vi "Swerve Calculate Angle and Velocity.vi"(4 "Max Translation Output(0-1)":dbl=1.0, 6 "Rotation Reduction":dbl=1.0, 7 "Frame":T1={"Length"=5.0, "Width"=1020.0}, 8 "Rotation Center From Robot Center":T2, 11 "Comand Data":T7 {"Rotate(Yaw) CCW 1 CW -1" scale=1.0..-1.0; "Traverse"."Angle" scale format="%.3f"; "Traverse"."Velocity" scale=-1.0..1.0 scale format="%.1f"}) -> (3 "Swerve Request Out":T3 {"Back Right"."Angle" scale format="%.3f"; "Back Right"."Velocity" scale=-1.0..1.0 scale format="%.1f"; "Back Left"."Angle" scale format="%.3f"; "Back Left"."Velocity" scale=-1.0..1.0 scale format="%.1f"; "Front Left"."Angle" scale format="%.3f"; "Front Left"."Velocity" scale=-1.0..1.0 scale format="%.1f"; "Front Right"."Angle" scale format="%.3f"; "Front Right"."Velocity" scale=-1.0..1.0 scale format="%.1f"})   [LabVIEW 2020, in "SwerveDrive_ACT.lvlib"]
doc: "Performs the kinematics for a rectangular four wheel swerve robot with a selectable center of rotation. Swerve module #0 is located in the front right corner and the modules increment in the counter-clockwise direction."
uses:
  SwerveDrive_ACT.lvlib
  Shared Code/TypeDefs/Cluster_CMD_Direction Data.ctl
  Shared Code/TypeDefs/Cluster_Module Velocity-Direction-Rotations.ctl
  Shared Code/TypeDefs/Level_Velocity plus-minus 1.ctl
  Shared Code/TypeDefs/Dial_Compase heading unit circle CCW positive.ctl
  Type Defs/NUM_Rotate Input.ctl
  Shared Code/TypeDefs/Cluster_Swerve 4 Steer and Velocity.ctl
  Shared Code/TypeDefs/Cluster_X-Y.ctl
  Type Defs/Cluster_Length and Width.ctl
panel:
  # "\"Front\" of Robot"
  # "Right Hand Rule"
  # "X"
  # "+CCW"
  # "Y"
  # "(0,0)"
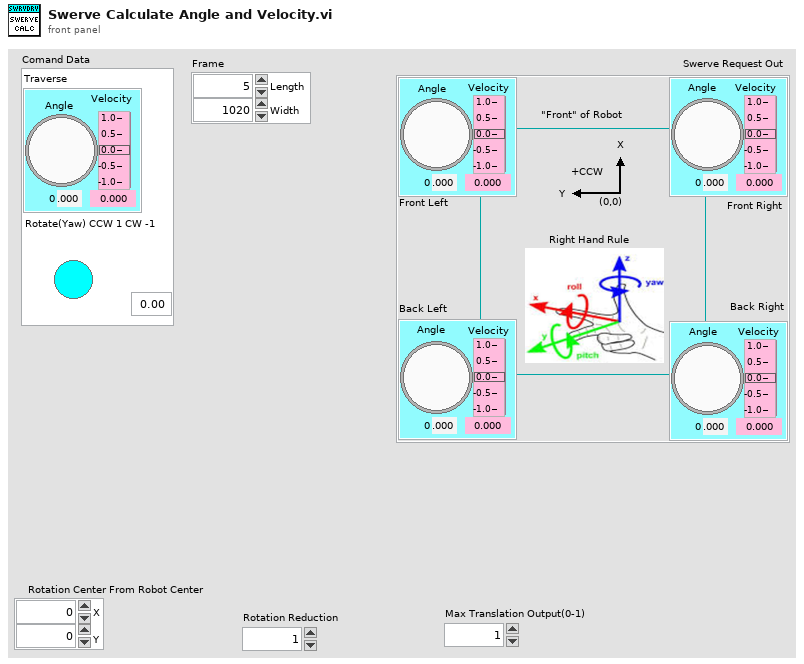
[diagram p1: front panel]
types:
  T1 = typedef "Cluster_Length and Width.ctl" = cluster{"Length":dbl, "Width":dbl}
  T2 = typedef "Cluster_X-Y.ctl" = cluster{"X":dbl, "Y":dbl}
  T3 = typedef "Cluster_Swerve 4 Steer and Velocity.ctl" = cluster{"Front Right":T4, "Front Left":T4, "Back Left":T4, "Back Right":T4}
  T4 = typedef "Cluster_Module Velocity-Direction-Rotations.ctl" = cluster{"Velocity":T5, "Angle":T6, "Rotations Count":dbl}
  T5 = typedef "Level_Velocity plus-minus 1.ctl" = dbl
  T6 = typedef "Dial_Compase heading unit circle CCW positive.ctl" = dbl
  T7 = typedef "Cluster_CMD_Direction Data.ctl" = cluster{"Traverse":T4, "Rotate(Yaw) CCW 1 CW -1":T8}
  T8 = typedef "NUM_Rotate Input.ctl" = dbl
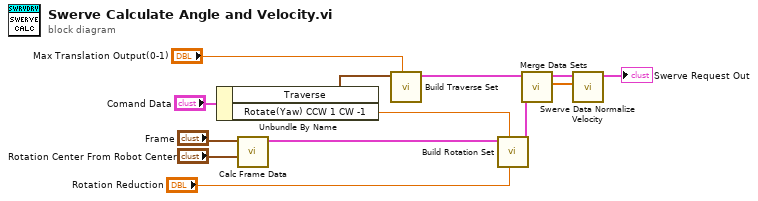
[diagram p0: block diagram]
diagram:
  n1 = Unbundle By Name("Comand Data") -> ("Traverse"=w4:T4, "Rotate(Yaw) CCW 1 CW -1"=w6:T8)
  n2 = call "Calc Frame Data .vi"("Rotation Center From Robot Center"="Rotation Center From Robot Center", "Frame"="Frame") -> ("Frame Rotation Set Out"=w5:T3)  [unwired: 9 in]
  n3 = call "Build Traverse Set.vi"("Max Translation Output(0-1)"="Max Translation Output(0-1)", "Traverse"=w4) -> ("Frame Rotation Set Out"=w7:T3)  [unwired: 9 in]
  n4 = call "Build Rotation Set.vi"("Rotation Reduction"="Rotation Reduction", "Rotate(Yaw) CCW 1 CW -1"=w6, "Frame Set"=w5) -> ("Rotation Set Out"=w3:T3)  [unwired: 8 in]
  n5 = call "Merge Data Sets.vi"("Rotation Set"=w3, "Traverse Set"=w7) -> ("Calcualted Velocities Out"=w11:dbl[], "Swerve Data Out"=w13:T3)  [unwired: 8 in]
  n6 = call "Swerve Data Normalize Velocity.vi"("Calcualted Velocities Out"=w11, "Swerve Data Out in"=w13) -> ("Swerve Data Out out"=→"Swerve Request Out":T3)  [unwired: 9 in]
